vi "Retrieve Data.vi"(8 "error in (no error)":errorcluster, 11 "Vaisala in":refnum<class "FPGA Vaisala.lvclass">) -> (0 "error out":errorcluster, 2 "Str Out":string, 3 "Vaisala out":refnum<class "FPGA Vaisala.lvclass">)   [LabVIEW 2015, in "FPGA Vaisala.lvclass"]
uses:
  FPGA Vaisala.lvclass
  FPGA Vaisala.lvclass/FPGA Vaisala.ctl
  <vilib>/Utility/error.llb/Error Cluster From Error Code.vi
  <vilib>/rvi/errors/niLvFpgaAdjustHostInterfaceError.vi
  <vilib>/RVI Host/nirviSupport.llb/nirviErrorClusterFromErrorCode.vi
  <vilib>/rvi/interface/nirviReadWriteControl/nirviReadWriteControl.xnode
  <vilib>/rvi/interface/nirviMethod/nirviMethod.xnode
  NiFpgaLv.dll
  <vilib>/FPGAPlugInAG/cRIO-9081/niLvFpga_AcknowledgeIrq_cRIO-9081.vi
  <vilib>/rvi/interface/nirviMethod/StockFPGA_InlinedMethodWaitForSingleIRQ.vi
  <vilib>/FPGAPlugInAG/cRIO-9081/niLvFpga_WaitOnIrq_cRIO-9081.vi
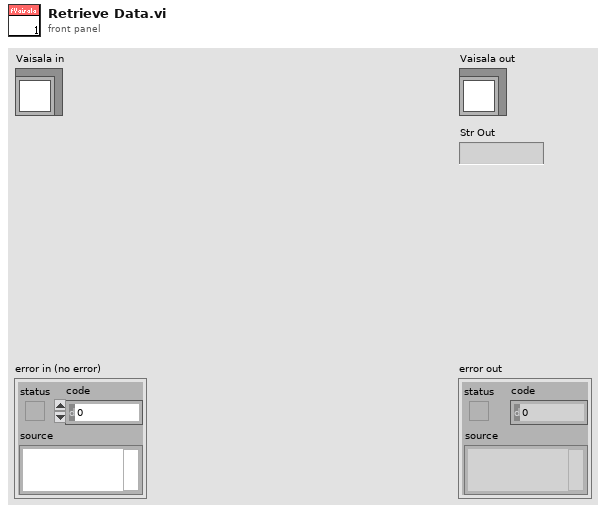
[diagram p1: front panel]
types:
  T1 = cluster{"Data":u8[], "NumBytes":i32, "RS485_Cmd":enum16{"Read", "Write", "Idle"}, "New":bool, "Port":enum16{"Port 1", "Port 2", "Port 3", "Port 4", "None"}, "Timeout (ms)":i32}
  T2 = enum16{"Port 1", "Port 2", "Port 3", "Port 4", "None"}
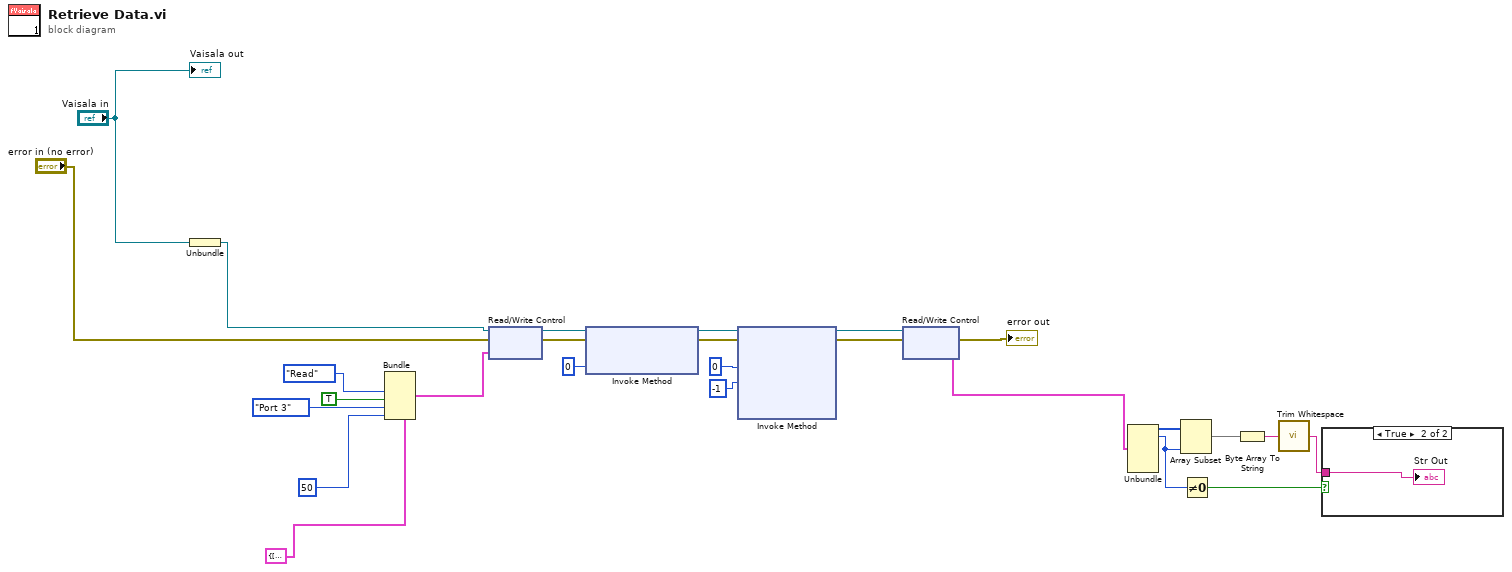
[diagram p0: block diagram]
diagram:
  n1 = Unbundle("Vaisala in") -> (w22:refnum<k20>)
  n2 = Bundle(cluster=T1 {"Data"=[0, 0, 0, 0, 0, 0, 0, 0, 0, 0, 0, 0, 0, 0, 0, 0, 0, 0, 0, 0, 0, 0, 0, 0, 0, 0, 0, 0, 0, 0, 0, 0, 0, 0, 0, 0, 0, 0, 0, 0, 0, 0, 0, 0, 0, 0, 0, 0, 0, 0, 0, 0, 0, 0, 0, 0, 0, 0, 0, 0, 0, 0, 0, 0, 0, 0, 0, 0, 0, 0, 0, 0, 0, 0, 0, 0, 0, 0, 0, 0, 0, 0, 0, 0, 0, 0, 0, 0, 0, 0, 0, 0, 0, 0, 0, 0, 0, 0, 0, 0], "NumBytes"=0, "RS485_Cmd"=enum."Read", "New"=FALSE, "Port"=enum."Port 1", "Timeout (ms)"=0} ("Input"), "RS485_Cmd"=enum16{"Read", "Write", "Idle"}."Read", "New"=TRUE ("New Message"), "Port"=T2."Port 3", "Timeout (ms)"=50) -> (w1:T1)  [unwired: 2 in]
  n3 = xnode "Read/Write Control"("FPGA VI Reference In"=w22, "error in"="error in (no error)", "Input"=w1) -> ("FPGA VI Reference Out"=w10:refnum<k20>, "error out"=w9:errorcluster)
  n4 = xnode "Invoke Method"("FPGA VI Reference In"=w10, "error in"=w9, "IRQ Number(s)"=0) -> ("FPGA VI Reference Out"=w14:refnum<k20>, "error out"=w13:errorcluster)
  n5 = xnode "Invoke Method"("FPGA VI Reference In"=w14, "error in"=w13, "IRQ Number(s)"=0, "Timeout (ms)"=-1) -> ("FPGA VI Reference Out"=w7:refnum<k20>, "error out"=w6:errorcluster)  [unwired: 2 out]
  n6 = xnode "Read/Write Control"("FPGA VI Reference In"=w7, "error in"=w6) -> ("error out"=→"error out":errorcluster, "Output"=w16:T1)  [unwired: 1 out]
  n7 = Unbundle(w16) -> ("Data"=w5:u8[], "NumBytes"=w4:i32)  [unwired: 4 out]
  n8 = Array Subset(array=w5, length=w4) -> (w18:u8[])  [unwired: 1 in]
  n9 = Not Equal To 0?(x=w4) -> (x != 0?=w17:bool)
  n10 = Byte Array To String(unsigned byte array=w18) -> (string=w20:string)
  n11 = call <vilib>:"Trim Whitespace.vi"("string"=w20) -> ("trimmed string"=w19:string)  [unwired: 1 in]
  n12 = case shown="True" w17 {
    tunnel: w19 -> [_ w27]
    frame False {
    }
    frame True {
      "Str Out" <- w27
    }
  }
  "Vaisala out" <- "Vaisala in"
